vi "Read CIPC Channel.vi"(8 "error in (no error)":errorcluster, 11 "CIFTag in":refnum<class "CIF_CIPC_Chn.lvclass">) -> (0 "error out":errorcluster, 2 "CIPC Channel":u64, 3 "CIFTag out":refnum<class "CIF_CIPC_Chn.lvclass">)   [LabVIEW 2021, in "CIF_CIPC_Chn.lvclass"]
uses:
  CIF_CIPC_Chn.lvclass
  CIF_CIPC_Chn.lvclass/CIF_CIPC_Chn.ctl
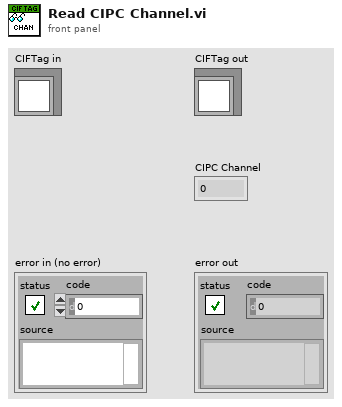
[diagram p1: front panel]
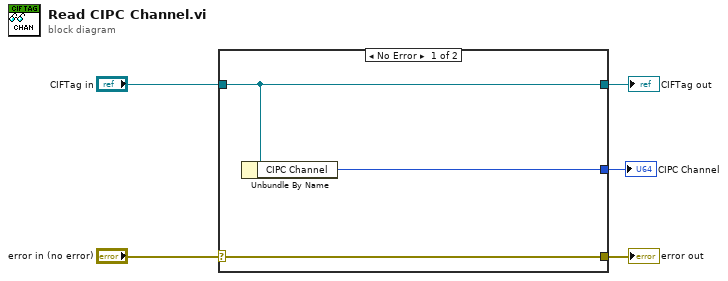
[diagram p0: block diagram]
diagram:
  n1 = case shown="No Error" "error in (no error)" {
    selector: "error in (no error)" -> [w8 w9]
    tunnel: [w8 w9] -> w4
    tunnel: [w7 w10] -> w2
    tunnel: "CIFTag in" -> [w7 w10]
    tunnel: [w6 _] -> w1
    frame No Error {
      n2 = Unbundle By Name(w7) -> ("CIPC Channel"=w6:u64)
    }
    frame Error {
    }
  }
  "error out" <- w4
  "CIFTag out" <- w2
  "CIPC Channel" <- w1
